vi "update_run_data.vi"(8 "error in":errorcluster, 10 "Run JSON":string, 11 "Run in":refnum<class "Run.lvclass">) -> (0 "error out":errorcluster, 3 "Run out":refnum<class "Run.lvclass">)   [LabVIEW 2020, in "Run.lvclass"]
uses:
  Run.lvclass
  Run Data.ctl
  Run.lvclass/Run.ctl
  6111fa5d-6312-4459-8f70-6676b09230da.vi
  7085f704-a81d-405d-a9ad-0f59f2d0802f.vi
  88df1df5-70e2-4e71-bcc4-80a84804b439.vi
  8f37e2be-7729-4acf-ba7c-a9ed101f2fc7.vi
  <vilib>/JDP Science/JSONtext/Find Item.vi
  <vilib>/JDP Science/JSONtext/Next JSON Value.vi
  <vilib>/JDP Science/JSONtext/String Subset.vi
  <vilib>/JDP Science/JSONtext/Parsing/Advance past next JSON Value (inlined COPY).vi
  <vilib>/JDP Science/JSONtext/Parsing/Advance past whitespace.vi
  <vilib>/JDP Science/JSONtext/Parsing/Advance past String.vi
  <vilib>/JDP Science/JSONtext/Parsing/Advance past Number.vi
  <vilib>/JDP Science/JSONtext/Parsing/Advance past Line Ending.vi
  <vilib>/JDP Science/JSONtext/Parsing/Parse Full Path or Item Name.vi
  <vilib>/JDP Science/JSONtext/Parsing/Advance past Array.vi
  <vilib>/JDP Science/JSONtext/Parsing/Advance past Object.vi
  <vilib>/JDP Science/JSONtext/support/Error Cluster From Code.vi
  <vilib>/JDP Science/JSONtext/Offset/Find Item Locations by Path.vi
  <vilib>/JDP Science/JSONtext/JSON text to Variant.vi
  <vilib>/JDP Science/JSONtext/LVClass Serializer/JSONtext LVClass Serializer.lvclass
  <vilib>/JDP Science/JSONtext/JSONtext.lvlib
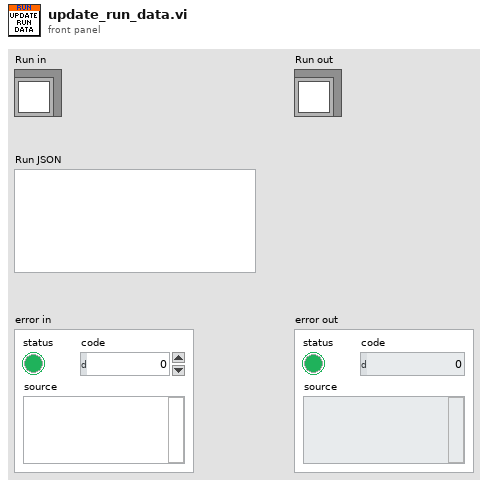
[diagram p1: front panel]
types:
  T1 = typedef "Run.lvclass/Run Data.ctl" = cluster{"rid":string, "runNumber":i32, "title":string, "description":string, "Run Properties":map{string, string}}
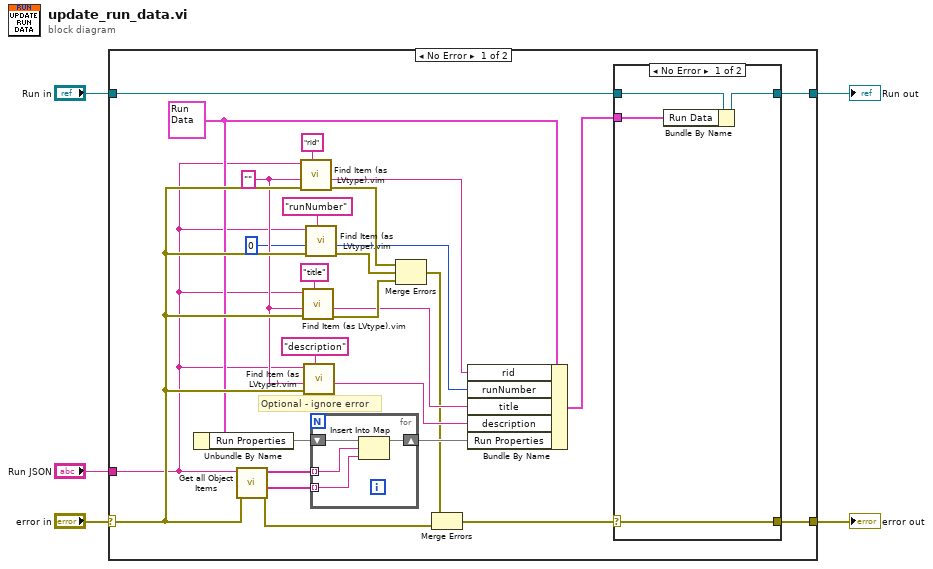
[diagram p0: block diagram]
diagram:
  n1 = case shown="No Error" "error in" {
    selector: "error in" -> [w32 w44]
    tunnel: "Run JSON" -> [w13 _]
    tunnel: "Run in" -> [w10 w43]
    tunnel: [w9 w43] -> w2
    tunnel: [w6 w44] -> w1
    frame No Error {
      w19 = "" ("$Path or Item Name")
      w28 = T1 {"rid"="", "runNumber"=0, "title"="", "description"="", "Run Properties"={}} ("Run Data")
      # "Optional - ignore error"
      n2 = Unbundle By Name(w28) -> ("Run Properties"=w29:map{string, string})
      n3 = call <vilib>:"Get all Object Items.vi"("error in (no error)"=w32, "JSON"=w13) -> ("error out"=w11:errorcluster, "<JSON>"=w30:string[], "Item Names"=w31:string[])  [unwired: 6 in, 1 out]
      n4 = call "Find Item (as LVtype).vim"("$Path or Item Name"="rid", "error in (no error)"=w32, "Data Type and Default Value"=w19, "JSON"=w13) -> ("error out"=w22:errorcluster, "Data"=w18:string)  [unwired: 4 in, 2 out]
      n5 = call "Find Item (as LVtype).vim"("$Path or Item Name"="title", "error in (no error)"=w32, "Data Type and Default Value"=w19, "JSON"=w13) -> ("error out"=w20:errorcluster, "Data"=w17:string)  [unwired: 4 in, 2 out]
      n6 = call "Find Item (as LVtype).vim"("$Path or Item Name"="description", "error in (no error)"=w32, "Data Type and Default Value"=w19, "JSON"=w13) -> ("Data"=w16:string)  [unwired: 4 in, 3 out]
      n7 = call "Find Item (as LVtype).vim"("$Path or Item Name"="runNumber", "error in (no error)"=w32, "Data Type and Default Value"=0, "JSON"=w13) -> ("error out"=w21:errorcluster, "Data"=w14:i32)  [unwired: 4 in, 2 out]
      n8 = for {
        tunnel: w31 -> [w42] mode=indexing
        tunnel: w30 -> [w41] mode=indexing
        shift-right: [w39] -> w27
        shift-left: w29 -> [w40]
        n9 = Insert Into Map(map in=w40, key=w42, value=w41) -> (map out=w39:map{string, string})  [unwired: 2 out]
      }
      n10 = Merge Errors(w22, w21, w20) -> (w12:errorcluster)
      n11 = Merge Errors(w12, w11) -> (w7:errorcluster)
      n12 = Bundle By Name(cluster=w28, "rid"=w18, "runNumber"=w14, "title"=w17, "description"=w16, "Run Properties"=w27) -> (w8:T1)
      n13 = case shown="No Error" w7 {
        selector: w7 -> [w33 w37]
        tunnel: w10 -> [w36 w38]
        tunnel: [w35 w38] -> w9
        tunnel: w8 -> [w34 _]
        tunnel: [w33 w37] -> w6
        frame No Error {
          n14 = Bundle By Name(cluster=w36, "Run Data"=w34) -> (w35:refnum<class "Run.lvclass">)
        }
        frame Error {
        }
      }
    }
    frame Error {
    }
  }
  "error out" <- w1
  "Run out" <- w2
